vi "PythonCaller.vi"() -> ()   [LabVIEW 2019]
uses:
  e185c1da-ac2d-4450-977a-4885e821bdf8.vi
  <vilib>/JDP Science/JSONtext/Variant to JSON Text.vi
  <vilib>/JDP Science/JSONtext/LVClass Serializer/JSONtext LVClass Serializer.lvclass
panel:
  in  "Tab Control":enum32{"Manual Control", "Automated PCR"}(tab)
  in  "Connect":bool
  in  "Enable Cmd":bool
  in  "Temperature Setpoint":dbl format="%.1g"
  in  "RunCycle":bool
  in  "nb_loops":u8=1 min=1 max=50 step=1
  out "error":errorcluster
  out "return value":string
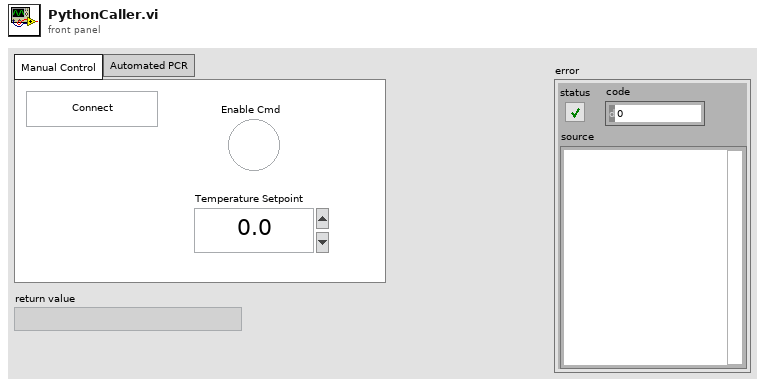
[diagram p1: front panel]
types:
  T1 = cluster{"appName":string, "remoteName":string, "mqtt-python":path, "Python session":refnum<k35>}
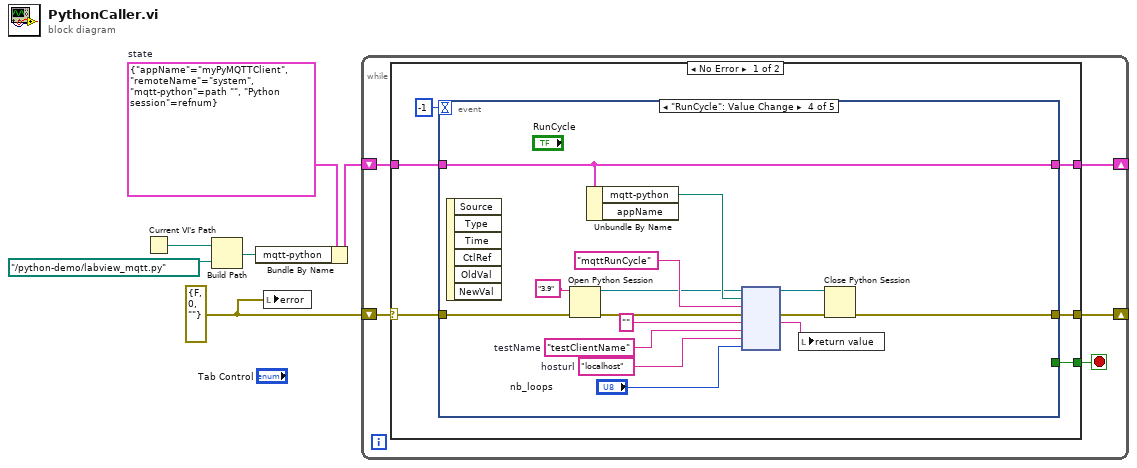
[diagram p0: block diagram]
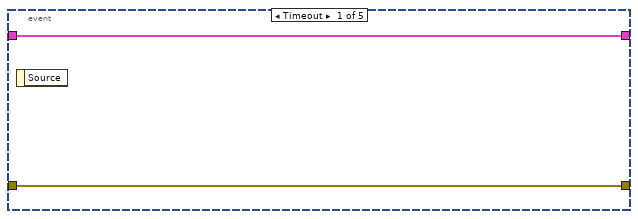
[diagram p2: hidden frame]
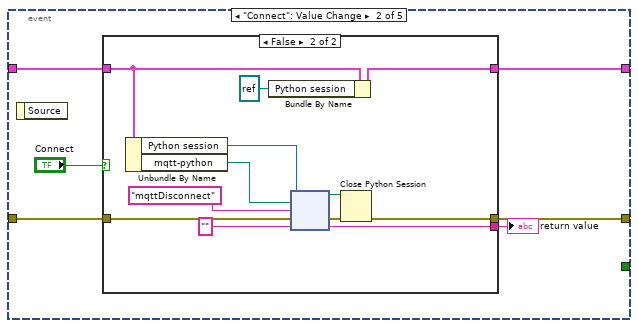
[diagram p3: hidden frame]
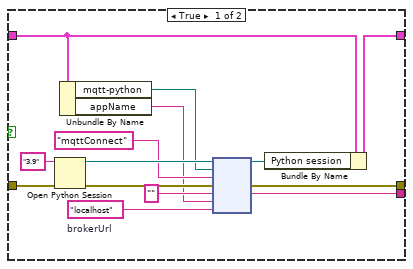
[diagram p4: hidden frame]
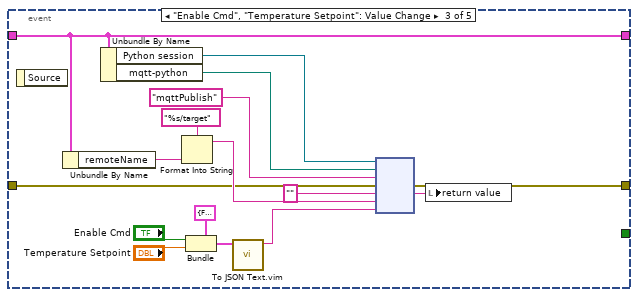
[diagram p5: hidden frame]
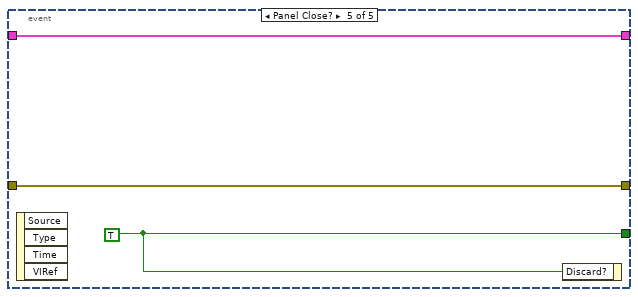
[diagram p6: hidden frame]
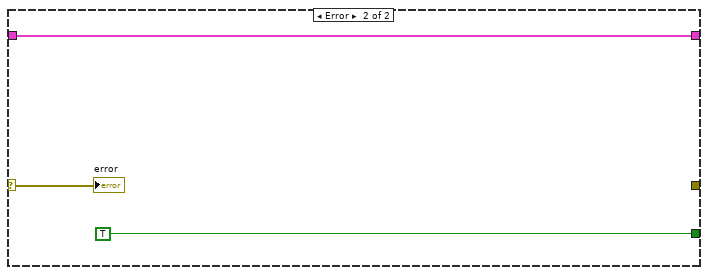
[diagram p7: hidden frame]
diagram:
  w1 = errorcluster {"status"=FALSE, "code"=0, "source"=""} ("error IO")
  w6 = T1 {"appName"="myPyMQTTClient", "remoteName"="system", "mqtt-python"=path "", "Python session"=refnum}  # state
  n1 = Current VI's Path() -> (path=w4:path)
  n2 = Build Path(base path=w4, name or relative path=path "../python-demo/labview_mqtt.py") -> (appended path=w2:path)
  n3 = Bundle By Name(cluster=w6, "mqtt-python"=w2) -> (w5:T1)
  n4 = local write "error"(w1) -> ()
  n5 = while {
    shift-right: [w11] -> _
    shift-left: w1 -> [w9]
    shift-right: [w7] -> _
    shift-left: w5 -> [w8]
    stop <- w10 stop-if-true
    n6 = case shown="No Error" w9 {
      selector: w9 -> [w14 w86]
      tunnel: [w17 _] -> w11
      tunnel: [w15 TRUE] -> w10
      tunnel: w8 -> [w13 w88]
      tunnel: [w12 w88] -> w7
      frame No Error {
        n7 = event shown="[3] \"RunCycle\": Value Change" {
          selector: _ -> [_ _ _ _ _]
          dyn-events: _ -> [_ _ _ _ _]
          timeout: -1 -> [_ _ _ _ _]
          tunnel: w14 -> [w18 w21 w52 w74 w84]
          tunnel: [w18 w22 w53 w70 w84] -> w17
          tunnel: [_ _ _ _ w85] -> w15
          tunnel: w13 -> [w19 w23 w62 w78 w83]
          tunnel: [w19 w24 w62 w78 w83] -> w12
          event Timeout {
            n8 = event-data() -> ()  [unwired: 1 in, 1 out]
          }
          event "Connect": Value Change {
            n9 = event-data() -> ()  [unwired: 1 in, 1 out]
            n10 = case shown="False" "Connect" {
              tunnel: [w34 w50] -> w25
              tunnel: [w30 w48] -> w24
              tunnel: w23 -> [w29 w47]
              tunnel: [w27 w40] -> w22
              tunnel: w21 -> [w26 w46]
              frame True {
                w33 = "localhost"  # brokerUrl
                n11 = Open Python Session(python version="3.9" ("Python version"), 3:w26) -> (session out=w38:refnum<k35>, error out=w37:errorcluster)  [unwired: 1 in]
                n12 = Unbundle By Name(w29) -> ("mqtt-python"=w32:path, "appName"=w28:string)
                n13 = node(w38, w32, "mqttConnect" ("Python version"), w37, "" ("Python version"), w28, w33) -> (w31:refnum<k35>, w27:errorcluster, w34:string)  [unwired: 2 in, 2 out]
                n14 = Bundle By Name(cluster=w29, "Python session"=w31) -> (w30:T1)
              }
              frame False {
                n15 = Unbundle By Name(w47) -> ("Python session"=w44:refnum<k35>, "mqtt-python"=w49:path)
                n16 = Bundle By Name(cluster=w47, "Python session"=refnum<k35> refnum) -> (w48:T1)
                n17 = node(w44, w49, "mqttDisconnect" ("Python version"), w46, "" ("Python version")) -> (w42:refnum<k35>, w41:errorcluster, w50:string)  [unwired: 2 out]
                n18 = Close Python Session(session in=w42, error in=w41) -> (11:w40:errorcluster)
              }
            }
            "return value" <- w25
          }
          event "Enable Cmd", "Temperature Setpoint": Value Change {
            n19 = event-data() -> ()  [unwired: 1 in, 1 out]
            n20 = Unbundle By Name(w62) -> ("remoteName"=w61:string)
            n21 = Unbundle By Name(w62) -> ("Python session"=w63:refnum<k35>, "mqtt-python"=w65:path)
            n22 = Format Into String(format string="%s/target", w61) -> (resulting string=w59:string)  [unwired: 2 in, 1 out]
            n23 = Bundle(cluster=cluster{"enable":bool, "setpoint":dbl} {"enable"=FALSE, "setpoint"=0.0}, "enable"="Enable Cmd", "setpoint"="Temperature Setpoint") -> (w55:cluster{"enable":bool, "setpoint":dbl})
            n24 = call "To JSON Text.vim"("Anything"=w55) -> ("<JSON>"=w54:string)  [unwired: 9 in, 1 out]
            n25 = node(w63, w65, "mqttPublish" ("Python version"), w52, "" ("Python version"), w59, w54) -> (w53:errorcluster, w64:string)  [unwired: 2 in, 3 out]
            n26 = local write "return value"(w64) -> ()
          }
          event "RunCycle": Value Change {
            w68 = "localhost"  # hosturl
            w69 = "testClientName"  # testName
            n27 = event-data() -> ()  [unwired: 1 in, 6 out]
            n28 = Open Python Session(python version="3.9" ("Python version"), 3:w74) -> (session out=w73:refnum<k35>, error out=w75:errorcluster)  [unwired: 1 in]
            n29 = Unbundle By Name(w78) -> ("mqtt-python"=w80:path)  [unwired: 1 out]
            n30 = node(w73, w80, "mqttRunCycle" ("Python version"), w75, "" ("Python version"), w69, w68, "nb_loops") -> (w72:refnum<k35>, w71:errorcluster, w79:string)  [unwired: 3 in, 2 out]
            n31 = local write "return value"(w79) -> ()
            n32 = Close Python Session(session in=w72, error in=w71) -> (11:w70:errorcluster)
          }
          event Panel Close? {
            w85 = TRUE
            n33 = event-data() -> ()  [unwired: 1 in, 4 out]
            n34 = event-data("Discard?"=w85) -> ()  [unwired: 1 in, 1 out]
          }
        }
      }
      frame Error {
        "error" <- w86
      }
    }
  }
